vi "Release-client-channel.vi"(8 "error in (no error)":errorcluster, 10 "Comm channel":refnum<queue>) -> (0 "error out":errorcluster)   [LabVIEW 2013, in "SLMServer.lvlib" / "SLMServer.lvclass"]
uses:
  SLMServer.lvclass
  SA-SLMAPI/Sources/Message.lvclass
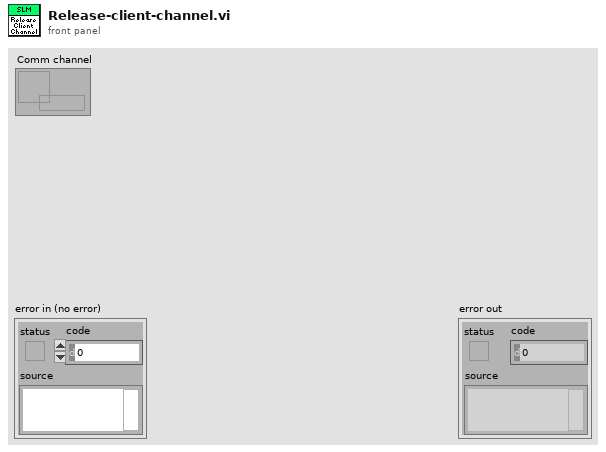
[diagram p1: front panel]
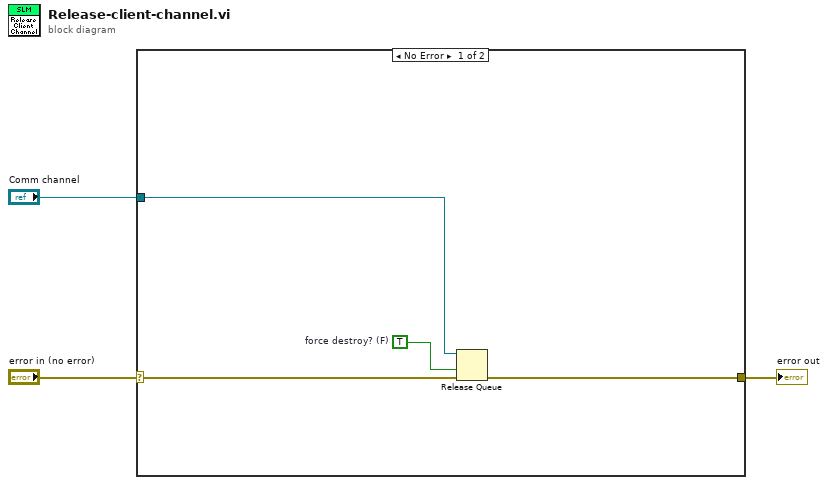
[diagram p0: block diagram]
diagram:
  n1 = case shown="No Error" "error in (no error)" {
    selector: "error in (no error)" -> [w7 w8]
    tunnel: [w6 w8] -> w2
    tunnel: "Comm channel" -> [w4 _]
    frame No Error {
      w5 = TRUE  # force destroy? (F)
      n2 = Release Queue(queue=w4, force destroy? (F)=w5, error in (no error)=w7) -> (error out=w6:errorcluster)  [unwired: 2 out]
    }
    frame Error {
    }
  }
  "error out" <- w2
